vi "In Range.vi"(9 "lower limit":u16, 10 "x":u16, 11 "upper limit":u16) -> (2 "in range":bool)   [LabVIEW 2016]
doc: "Checks if x is bigger or equal to lower limit and lower then upper limit."
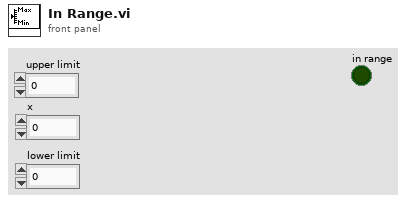
[diagram p1: front panel]
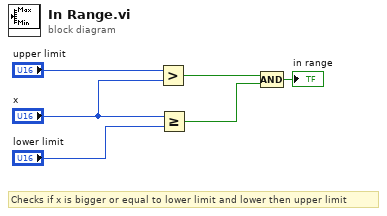
[diagram p0: block diagram]
diagram:
  # "Checks if x is bigger or equal to lower limit and lower then upper limit"
  n1 = Greater?(x="upper limit", y="x") -> (0:w3:bool)
  n2 = Greater Or Equal?(x="x", y="lower limit") -> (x >= y?=w2:bool)
  n3 = Compound Arithmetic op=AND(w3, w2) -> (→"in range":bool)
